vi "Send Data to FPGA.vi"(8 "error in (no error)":errorcluster, 9 "Data":variant, 11 "Command":string) -> (0 "error out":errorcluster)   [LabVIEW 2024, in "FPGA Interface.lvlib"]
uses:
  FPGA Interface.lvlib
  Shared Modules/CAN Commands Interpreter/Command Values.ctl
  FPGA Reference - Get.vi
  <vilib>/Utility/error.llb/Error Cluster From Error Code.vi
  <vilib>/rvi/errors/niLvFpgaAdjustHostInterfaceError.vi
  <vilib>/rvi/Analysis/host/Private/Sample Rate To Loop Time (ticks).vi
  <vilib>/RVI Host/nirviSupport.llb/nirviErrorClusterFromErrorCode.vi
  Type Definitions/ECU FPGA Reference.ctl
  <vilib>/rvi/interface/nirviReadWriteControl/nirviReadWriteControl.xnode
  FPGA Bitfiles/ecu-9030_FPGATarget_FPGAMain_pDLqQGhG1UY.lvbitx
  <vilib>/rvi/interface/nirviMethod/nirviMethod.xnode
  NiFpgaLv.dll
  Real-Time ECU/RT Management.lvlib
  <vilib>/rvi/Analysis/host/Public/NI_FpgaMspHost.lvlib
  Shared Modules/CAN Commands Interpreter/CAN Commands.lvlib
  <vilib>/rvi/interface/nirviMethod/StockFPGA_InlinedMethodWaitForSingleIRQ.vi
  <vilib>/FPGAPlugInAG/cRIO-9030/niLvFpga_WaitOnIrq_cRIO-9030.vi
  <vilib>/FPGAPlugInAG/cRIO-9030/niLvFpga_AcknowledgeIrq_cRIO-9030.vi
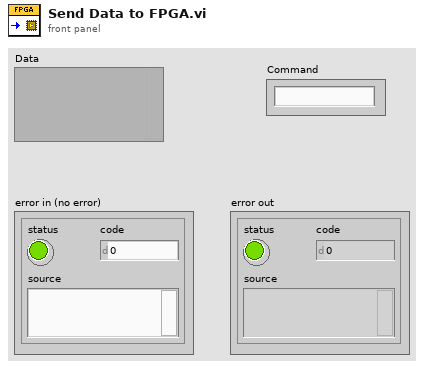
[diagram p1: front panel]
types:
  T1 = cluster{"Frequency (periods/tick)":fxp<+,32,0>, "Phase offset (periods)":fxp<+,32,0>, "duty cycle (periods)":fxp<+,32,0>}
  T2 = cluster{"Frequency (periods/tick)":fxp<+,32,0>, "Phase offset (periods)":fxp<+,32,0>, "Scale factor":fxp<+/-,16,1>, "Amplitude offset":fxp<+/-,16,16>}
  T3 = typedef "CAN Commands.lvlib/Command Values.ctl" = cluster{"Command":string, "Value":dbl}
  T4 = typedef "ECU FPGA Reference.ctl" = refnum<k20>
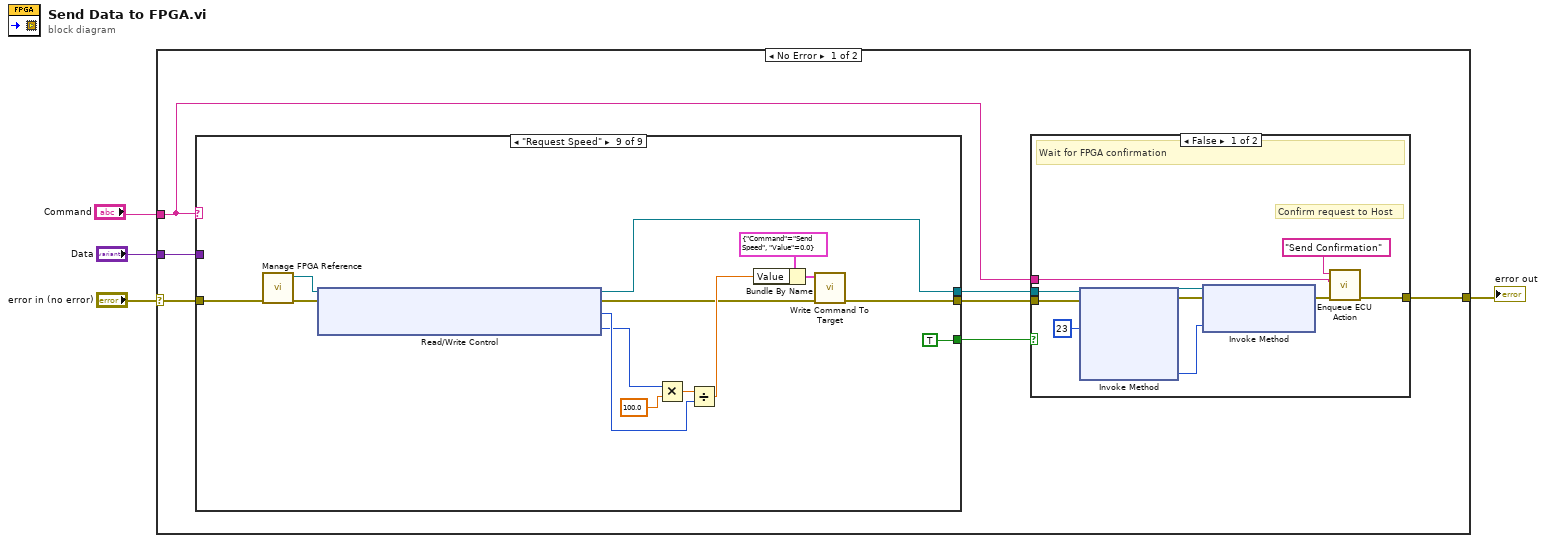
[diagram p0: block diagram]
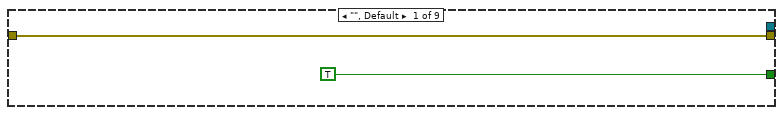
[diagram p2: hidden frame]
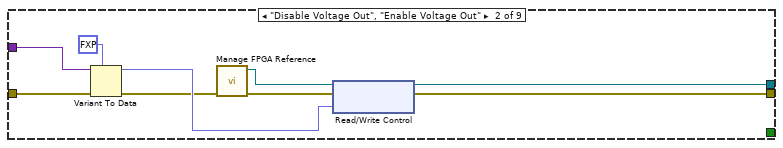
[diagram p3: hidden frame]
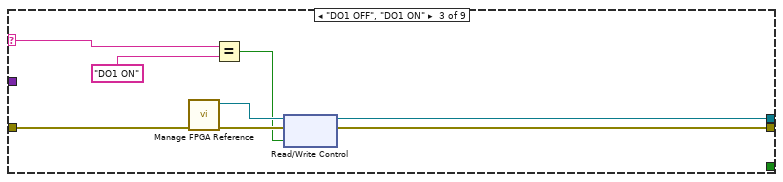
[diagram p4: hidden frame]
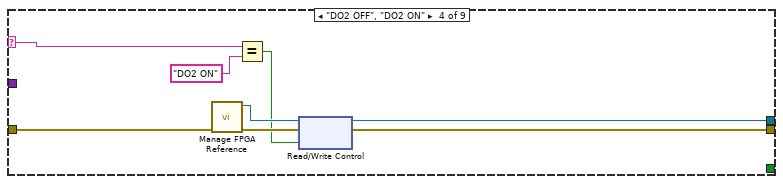
[diagram p5: hidden frame]
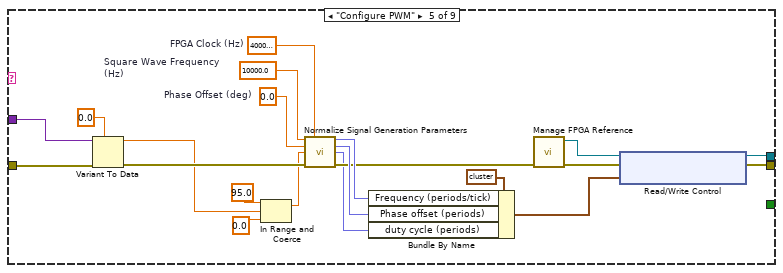
[diagram p6: hidden frame]
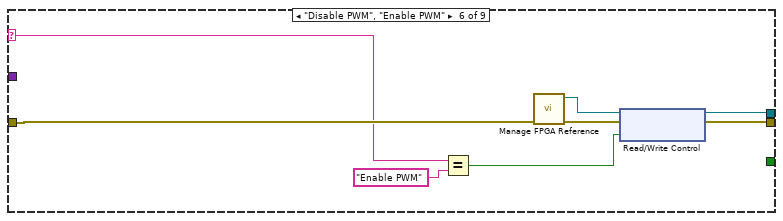
[diagram p7: hidden frame]
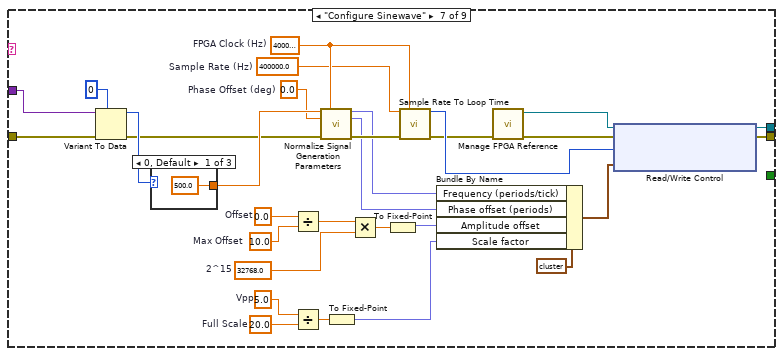
[diagram p8: hidden frame]
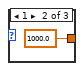
[diagram p9: hidden frame]
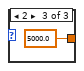
[diagram p10: hidden frame]
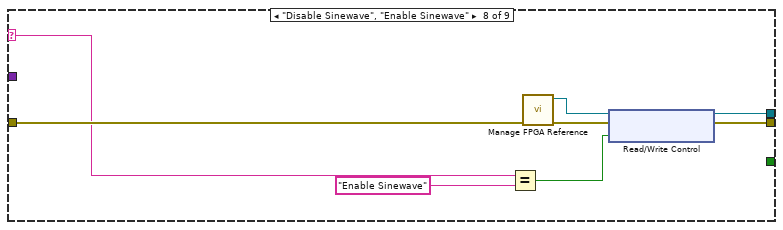
[diagram p11: hidden frame]
diagram:
  n1 = case shown="No Error" "error in (no error)" {
    selector: "error in (no error)" -> [w7 w134]
    tunnel: "Data" -> [w11 _]
    tunnel: [w6 w134] -> w3
    tunnel: "Command" -> [w5 _]
    frame No Error {
      n2 = case shown="\"Request Speed\"" w5 {
        selector: w5 -> [_ _ w26 w32 _ w62 _ w101 _]
        tunnel: w11 -> [_ w21 _ _ w56 _ w71 _ _]
        tunnel: w7 -> [w13 w18 w25 w33 w57 w65 w72 w104 w112]
        tunnel: [w13 w17 w24 w34 w54 w64 w74 w102 w111] -> w10
        tunnel: [_ w14 w23 w31 w44 w63 w75 w103 w110] -> w9
        tunnel: [TRUE _ _ _ _ _ _ _ TRUE] -> w8
        frame "", Default {
        }
        frame "Disable Voltage Out", "Enable Voltage Out" {
          n3 = Variant To Data(error in=w18, type=fxp<+/-,20,5> 0.0 ("Voltage Out"), Variant=w21) -> (data=w22:fxp<+/-,20,5>, error out=w19:errorcluster)
          n4 = call-poly "Manage FPGA Reference.vi"("error in"=w19) -> ("error out"=w15:errorcluster, "FPGA Reference Out"=w16:T4)  [unwired: 9 in]
          n5 = xnode "Read/Write Control"("FPGA VI Reference In"=w16, "error in"=w15, "Voltage Out"=w22) -> ("FPGA VI Reference Out"=w14:T4, "error out"=w17:errorcluster)
        }
        frame "DO1 OFF", "DO1 ON" {
          n6 = call-poly "Manage FPGA Reference.vi"("error in"=w25) -> ("error out"=w29:errorcluster, "FPGA Reference Out"=w30:T4)  [unwired: 9 in]
          n7 = Equal?(x=w26, y="DO1 ON") -> (x = y?=w27:bool)
          n8 = xnode "Read/Write Control"("FPGA VI Reference In"=w30, "error in"=w29, "DO1"=w27) -> ("FPGA VI Reference Out"=w23:T4, "error out"=w24:errorcluster)
        }
        frame "DO2 OFF", "DO2 ON" {
          n9 = call-poly "Manage FPGA Reference.vi"("error in"=w33) -> ("error out"=w37:errorcluster, "FPGA Reference Out"=w38:T4)  [unwired: 9 in]
          n10 = Equal?(x=w32, y="DO2 ON") -> (x = y?=w36:bool)
          n11 = xnode "Read/Write Control"("FPGA VI Reference In"=w38, "error in"=w37, "DO2"=w36) -> ("FPGA VI Reference Out"=w31:T4, "error out"=w34:errorcluster)
        }
        frame "Configure PWM" {
          w48 = 10000.0  # Square Wave Frequency (Hz)
          w51 = 40000000.0  # FPGA Clock (Hz)
          w50 = 0.0  # Phase Offset (deg)
          n12 = Variant To Data(error in=w57, type=0.0, Variant=w56) -> (data=w42:dbl, error out=w47:errorcluster)
          n13 = In Range and Coerce(upper limit=95.0, x=w42, lower limit=0.0) -> (coerced(x)=w39:dbl)  [unwired: 1 out]
          n14 = call <vilib>:"Normalize Signal Generation Parameters.vi"("frequency (Hz)"=w48, "FPGA clock rate (Hz)"=w51, "phase offset (deg)"=w50, "duty cycle (%)"=w39, "error in (no error)"=w47) -> ("frequency (periods/tick)"=w53:fxp<+,32,0>, "phase offset (periods)"=w52:fxp<+,32,0>, "duty cycle (periods)"=w43:fxp<+,32,0>, "error out"=w46:errorcluster)  [unwired: 5 in, 2 out]
          n15 = Bundle By Name(cluster=T1 {"Frequency (periods/tick)"=0.9999999997671694, "Phase offset (periods)"=0.0, "duty cycle (periods)"=0.0} ("Square Wave Settings"), "Frequency (periods/tick)"=w53, "Phase offset (periods)"=w52, "duty cycle (periods)"=w43) -> (w45:T1)
          n16 = call-poly "Manage FPGA Reference.vi"("error in"=w46) -> ("error out"=w58:errorcluster, "FPGA Reference Out"=w59:T4)  [unwired: 9 in]
          n17 = xnode "Read/Write Control"("FPGA VI Reference In"=w59, "error in"=w58, "Squarewave Settings"=w45) -> ("FPGA VI Reference Out"=w44:T4, "error out"=w54:errorcluster)
        }
        frame "Disable PWM", "Enable PWM" {
          n18 = Equal?(x=w62, y="Enable PWM") -> (x = y?=w60:bool)
          n19 = call-poly "Manage FPGA Reference.vi"("error in"=w65) -> ("error out"=w66:errorcluster, "FPGA Reference Out"=w67:T4)  [unwired: 9 in]
          n20 = xnode "Read/Write Control"("FPGA VI Reference In"=w67, "error in"=w66, "Enable PWM"=w60) -> ("FPGA VI Reference Out"=w63:T4, "error out"=w64:errorcluster)
        }
        frame "Configure Sinewave" {
          w77 = 0.0  # Phase Offset (deg)
          w76 = 400000.0  # Sample Rate (Hz)
          w82 = 0.0  # Offset
          w80 = 5.0  # Vpp
          w78 = 40000000.0  # FPGA Clock (Hz)
          w83 = 10.0  # Max Offset
          w84 = 32768.0  # 2^15
          w81 = 20.0  # Full Scale
          n21 = Variant To Data(error in=w72, type=u8 0, Variant=w71) -> (data=w70:u8, error out=w69:errorcluster)
          n22 = case shown="0, Default" w70 {
            tunnel: [500.0 ("Voffset (V)") 1000.0 ("Voffset (V)") 5000.0 ("Voffset (V)")] -> w91
            frame 0, Default {
            }
            frame 1 {
            }
            frame 2 {
            }
          }
          n23 = Divide(x=w82, y=w83) -> (x/y=w89:dbl)
          n24 = Divide(x=w80, y=w81) -> (x/y=w88:dbl)
          n25 = call <vilib>:"Normalize Signal Generation Parameters.vi"("frequency (Hz)"=w91, "FPGA clock rate (Hz)"=w78, "phase offset (deg)"=w77, "error in (no error)"=w69) -> ("frequency (periods/tick)"=w85:fxp<+,32,0>, "phase offset (periods)"=w86:fxp<+,32,0>, "error out"=w90:errorcluster)  [unwired: 6 in, 3 out]
          n26 = To Fixed-Point(number=w88) -> (fixed-point=w68:fxp<+/-,16,1>)  [unwired: 1 in]
          n27 = Multiply(x=w89, y=w84) -> (x*y=w87:dbl)
          n28 = To Fixed-Point(number=w87) -> (fixed-point=w92:fxp<+/-,16,16>)  [unwired: 1 in]
          n29 = call-poly <vilib>:"Sample Rate To Loop Time.vi"("sample rate (S/s)"=w76, "FPGA clock rate (Hz)"=w78, "error in (no error)"=w90) -> ("count (ticks/S)"=w97:u32, "error out"=w95:errorcluster)  [unwired: 10 in, 1 out]
          n30 = Bundle By Name(cluster=T2 {"Frequency (periods/tick)"=0.0, "Phase offset (periods)"=0.0, "Scale factor"=0.999969482421875, "Amplitude offset"=0.0} ("Sinewave Props 0"), "Frequency (periods/tick)"=w85, "Phase offset (periods)"=w86, "Amplitude offset"=w92, "Scale factor"=w68) -> (w96:T2)
          n31 = call-poly "Manage FPGA Reference.vi"("error in"=w95) -> ("error out"=w93:errorcluster, "FPGA Reference Out"=w94:T4)  [unwired: 9 in]
          n32 = xnode "Read/Write Control"("FPGA VI Reference In"=w94, "error in"=w93, "Desired loop rate (ticks)"=w97, "Sinewave Settings"=w96) -> ("FPGA VI Reference Out"=w75:T4, "error out"=w74:errorcluster)
        }
        frame "Disable Sinewave", "Enable Sinewave" {
          n33 = Equal?(x=w101, y="Enable Sinewave") -> (x = y?=w106:bool)
          n34 = call-poly "Manage FPGA Reference.vi"("error in"=w104) -> ("error out"=w107:errorcluster, "FPGA Reference Out"=w108:T4)  [unwired: 9 in]
          n35 = xnode "Read/Write Control"("FPGA VI Reference In"=w108, "error in"=w107, "Enable Sinewave"=w106) -> ("FPGA VI Reference Out"=w103:T4, "error out"=w102:errorcluster)
        }
        frame "Request Speed" {
          n36 = call-poly "Manage FPGA Reference.vi"("error in"=w112) -> ("error out"=w116:errorcluster, "FPGA Reference Out"=w115:T4)  [unwired: 9 in]
          n37 = xnode "Read/Write Control"("FPGA VI Reference In"=w115, "error in"=w116) -> ("FPGA VI Reference Out"=w110:T4, "error out"=w121:errorcluster, "Period (Ticks)"=w118:u32, "High Period (Ticks)"=w113:u32)
          n38 = Multiply(x=w113, y=100.0) -> (x*y=w114:dbl)
          n39 = Divide(x=w114, y=w118) -> (x/y=w122:dbl)
          n40 = Bundle By Name(cluster=T3 {"Command"="Send Speed", "Value"=0.0} ("Command"), "Value"=w122) -> (w120:T3)
          n41 = call "Write Command To Target.vi"("error out"=w121, "Command"=w120) -> ("error out"=w111:errorcluster)  [unwired: 9 in]
        }
      }
      n42 = case shown="False" w8 {
        tunnel: w10 -> [w128 w133]
        tunnel: w9 -> [w127 _]
        tunnel: [w126 w133] -> w6
        tunnel: w5 -> [w124 _]
        frame False {
          # "Confirm request to Host"
          # "Wait for FPGA confirmation"
          n43 = xnode "Invoke Method"("FPGA VI Reference In"=w127, "error in"=w128, "IRQ Number(s)"=23) -> ("FPGA VI Reference Out"=w131:T4, "error out"=w130:errorcluster, "IRQ(s) Asserted"=w132:i32)  [unwired: 1 in, 1 out]
          n44 = xnode "Invoke Method"("FPGA VI Reference In"=w131, "error in"=w130, "IRQ Number(s)"=w132) -> ("error out"=w125:errorcluster)  [unwired: 1 out]
          n45 = call "Enqueue ECU Action.vi"("error in"=w125, "Command"=w124, "Message"="Send Confirmation") -> ("error out"=w126:errorcluster)  [unwired: 8 in]
        }
        frame True {
        }
      }
    }
    frame Error {
    }
  }
  "error out" <- w3
